vi "Relative Path String To Array Of Strings.vi"(11 "Relative Path":string) -> (3 "Relative Path Array":string[](array[string]))   [LabVIEW 2011, in "LMH-Toolbox.lvlib" / "LMH-Common.lvlib"]
doc: "Convert a relative path into a string array. This is useful for removeing platform dependent slashes from relative paths."
uses:
  LMH-Common.lvlib
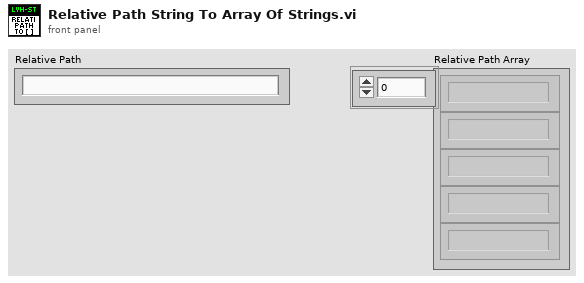
[diagram p1: front panel]
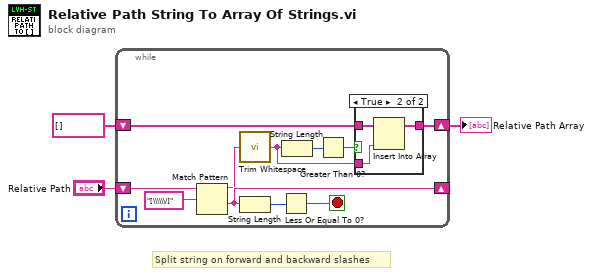
[diagram p0: block diagram]
diagram:
  # "Split string on forward and backward slashes"
  n1 = while {
    shift-right: [w10] -> _
    shift-left: "Relative Path" -> [w12]
    shift-right: [w13] -> w1
    shift-left: string[] [] -> [w14]
    stop <- w8 stop-if-true
    n2 = Match Pattern(string=w12, regular expression="[\\\\\\/]") -> (before substring=w7:string, after substring=w10:string)  [unwired: 1 in, 2 out]
    n3 = call <vilib>:"Trim Whitespace.vi"("string"=w7) -> ("trimmed string"=w4:string)  [unwired: 1 in]
    n4 = String Length(string=w10) -> (length=w9:i32)
    n5 = Less Or Equal To 0?(x=w9) -> (x <= 0?=w8:bool)
    n6 = String Length(string=w4) -> (length=w6:i32)
    n7 = Greater Than 0?(x=w6) -> (x > 0?=w5:bool)
    n8 = case shown="True" w5 {
      tunnel: w14 -> [w15 w18]
      tunnel: [w15 w17] -> w13
      tunnel: w4 -> [_ w16]
      frame False {
      }
      frame True {
        n9 = Insert Into Array(array=w18, new element=w16) -> (w17:string[])  [unwired: 1 in]
      }
    }
  }
  "Relative Path Array" <- w1
